vi "Obtain Reentrant VI Name.vi"(10 "error in (no error)":errorcluster, 11 "Call Depth (1)":i32=1) -> (2 "error out":errorcluster, 3 "Clone Name":string)   [LabVIEW 2020, in "Dynamic Reentrant.lvlib"]
uses:
  <userlib>/Dynamic Reentrant/Dynamic Reentrant.lvlib
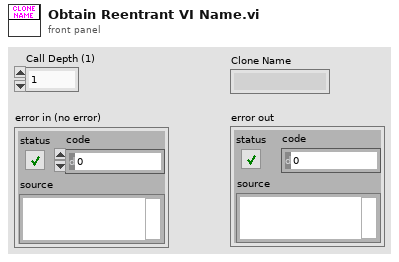
[diagram p1: front panel]
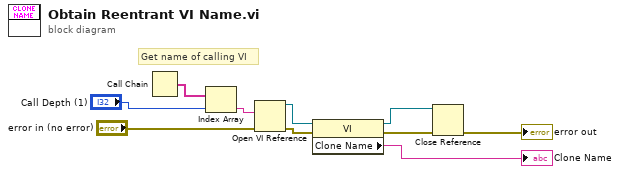
[diagram p0: block diagram]
diagram:
  # "Get name of calling VI"
  n1 = Call Chain() -> (call chain=w9:string[])
  n2 = Index Array(array=w9, index="Call Depth (1)") -> (element=w7:string)
  n3 = Open VI Reference(vi path=w7, error in (no error)="error in (no error)") -> (vi reference=w5:refnum<vi>, error out=w6:errorcluster)  [unwired: 4 in]
  n4 = property class="VI"(reference=w5, error in=w6) -> (reference out=w4:refnum<vi>, error out=w3:errorcluster, "Clone Name"=→"Clone Name":string)
  n5 = Close Reference(reference=w4, error in (no error)=w3) -> (error out=→"error out":errorcluster)
